vi "In Range.vi"(9 "Array":cluster{i64, i64, i64}[](array[cluster]), 10 "Min Range":cluster{i64, i64, i64}, 11 "Max Range":cluster{i64, i64, i64}) -> (3 "Boolean":bool)   [LabVIEW 2021, in "d18.lvlib"]
uses:
  d18.lvlib
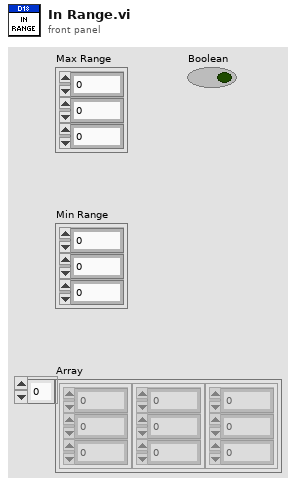
[diagram p1: front panel]
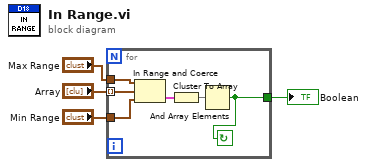
[diagram p0: block diagram]
diagram:
  n1 = for {
    tunnel: "Array" -> [w10] mode=indexing
    tunnel: "Max Range" -> [w9]
    tunnel: "Min Range" -> [w8]
    tunnel: [w5] -> w1
    stop <- w5 continue-if-true
    n2 = In Range and Coerce(upper limit=w9, x=w10, lower limit=w8) -> (In Range?=w7:cluster{bool, bool, bool})  [unwired: 1 out]
    n3 = Cluster To Array(cluster=w7) -> (array=w6:bool[])
    n4 = And Array Elements(Boolean array=w6) -> (logical AND=w5:bool)
  }
  "Boolean" <- w1
